vi "WriteEnvironmentInfo.vi"(4 "error in (no error)":errorcluster, 5 "# of Entries (before)":i16, 6 "EnvironmentalInfo":T1, 7 "Pathto FITS Header File":path) -> (0 "error out":errorcluster, 2 "# of Entries (after)":i16, 3 "Path to FITS Header File":path)   [LabVIEW 2015]
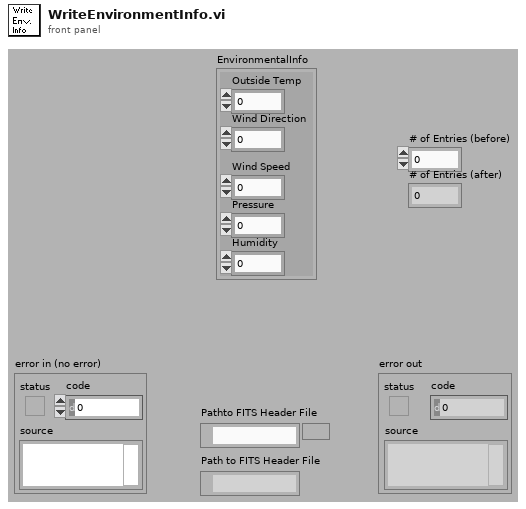
[diagram p1: front panel]
types:
  T1 = cluster{"Outside Temp":dbl, "Wind Direction":dbl, "Wind Speed":dbl, "Pressure":dbl, "Humidity":dbl}
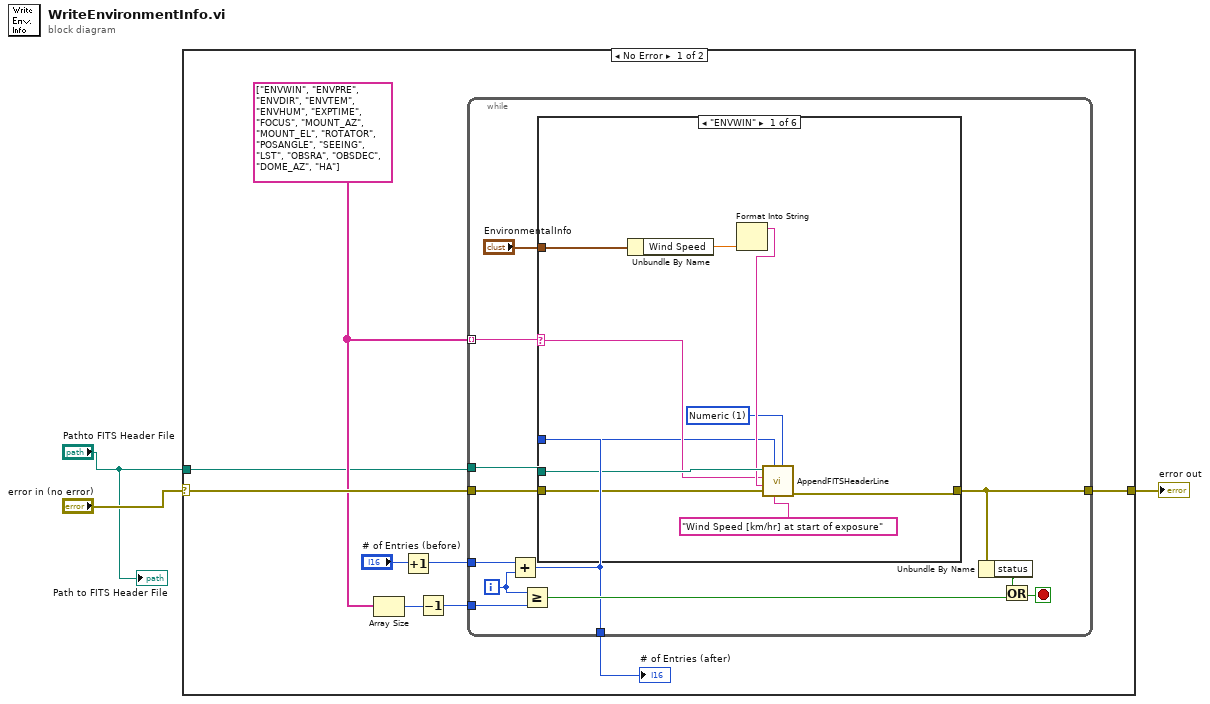
[diagram p0: block diagram]
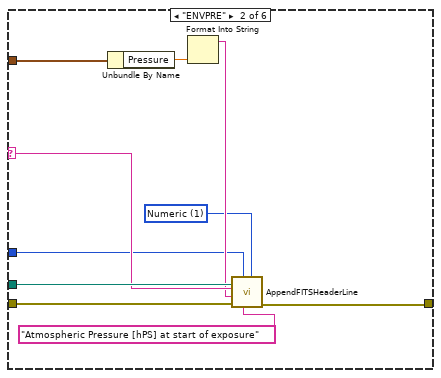
[diagram p2: hidden frame]
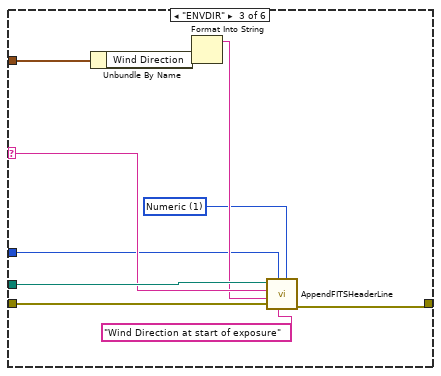
[diagram p3: hidden frame]
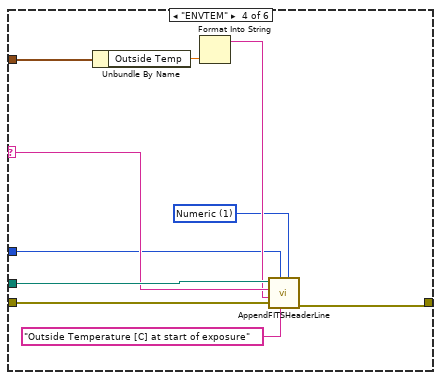
[diagram p4: hidden frame]
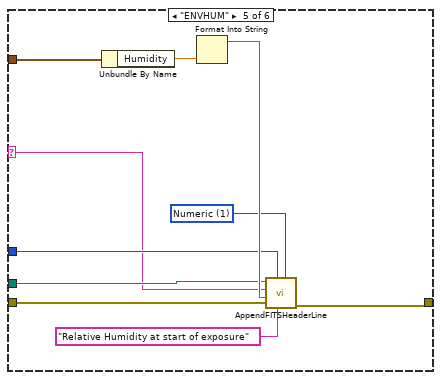
[diagram p5: hidden frame]
diagram:
  n1 = case shown="No Error" "error in (no error)" {
    selector: "error in (no error)" -> [w12 w76]
    tunnel: [w8 w76] -> w2
    tunnel: "Pathto FITS Header File" -> [w7 _]
    frame No Error {
      w11 = string[] ["ENVWIN", "ENVPRE", "ENVDIR", "ENVTEM", "ENVHUM", "EXPTIME", "FOCUS", "MOUNT_AZ", "MOUNT_EL", "ROTATOR", "POSANGLE", "SEEING", "LST", "OBSRA", "OBSDEC", "DOME_AZ", "HA"]
      n2 = Array Size(array=w11) -> (size(s)=w10:i32)
      n3 = Increment(x="# of Entries (before)") -> (x+1=w5:i16)
      n4 = Decrement(x=w10) -> (x-1=w9:i32)
      n5 = while {
        tunnel: w12 -> [w24]
        tunnel: w11 -> [w21] mode=indexing
        tunnel: w9 -> [w20]
        tunnel: [w19] -> w8
        tunnel: w7 -> [w16]
        tunnel: w5 -> [w14]
        tunnel: [w13] -> w4
        i -> [w15]
        stop <- w23 stop-if-true
        n6 = Add(x=w14, y=w15) -> (x+y=w13:i32)
        n7 = Greater Or Equal?(x=w15, y=w20) -> (x >= y?=w18:bool)
        n8 = case shown="\"ENVWIN\"" w21 {
          selector: w21 -> [w28 w40 w49 w59 w66 _]
          tunnel: w24 -> [w32 w43 w52 w62 w69 w75]
          tunnel: [w31 w42 w51 w61 w70 w75] -> w19
          tunnel: "EnvironmentalInfo" -> [w34 w44 w54 w64 w65 _]
          tunnel: w16 -> [w30 w41 w50 w60 w68 _]
          tunnel: w13 -> [w27 w37 w46 w57 w67 _]
          frame "ENVWIN" {
            w26 = u16 1 items=["String", "Numeric", "Boolean"] ("Entry Type")
            n9 = Unbundle By Name(w34) -> ("Wind Speed"=w33:dbl)
            n10 = Format Into String(w33) -> (resulting string=w29:string)  [unwired: 3 in, 1 out]
            n11 = call "AppendFITSHeaderLine.vi"("Entry Type"=w26, "Comment"="Wind Speed [km/hr] at start of exposure", "Entry #"=w27, "error in (no error)"=w32, "Element Value"=w29, "Element Name"=w28, "file path (dialog if empty)"=w30) -> ("error out"=w31:errorcluster)  [unwired: 3 in]
          }
          frame "ENVPRE" {
            w36 = u16 1 items=["String", "Numeric", "Boolean"] ("Entry Type")
            n12 = Unbundle By Name(w44) -> ("Pressure"=w39:dbl)
            n13 = Format Into String(w39) -> (resulting string=w38:string)  [unwired: 3 in, 1 out]
            n14 = call "AppendFITSHeaderLine.vi"("Entry Type"=w36, "Comment"="Atmospheric Pressure [hPS] at start of exposure", "Entry #"=w37, "error in (no error)"=w43, "Element Value"=w38, "Element Name"=w40, "file path (dialog if empty)"=w41) -> ("error out"=w42:errorcluster)  [unwired: 3 in]
          }
          frame "ENVDIR" {
            w47 = u16 1 items=["String", "Numeric", "Boolean"] ("Entry Type")
            n15 = Unbundle By Name(w54) -> ("Wind Direction"=w53:dbl)
            n16 = Format Into String(w53) -> (resulting string=w48:string)  [unwired: 3 in, 1 out]
            n17 = call "AppendFITSHeaderLine.vi"("Entry Type"=w47, "Comment"="Wind Direction at start of exposure", "Entry #"=w46, "error in (no error)"=w52, "Element Value"=w48, "Element Name"=w49, "file path (dialog if empty)"=w50) -> ("error out"=w51:errorcluster)  [unwired: 3 in]
          }
          frame "ENVTEM" {
            w56 = u16 1 items=["String", "Numeric", "Boolean"] ("Entry Type")
            n18 = Unbundle By Name(w64) -> ("Outside Temp"=w63:dbl)
            n19 = Format Into String(w63) -> (resulting string=w58:string)  [unwired: 3 in, 1 out]
            n20 = call "AppendFITSHeaderLine.vi"("Entry Type"=w56, "Comment"="Outside Temperature [C] at start of exposure", "Entry #"=w57, "error in (no error)"=w62, "Element Value"=w58, "Element Name"=w59, "file path (dialog if empty)"=w60) -> ("error out"=w61:errorcluster)  [unwired: 3 in]
          }
          frame "ENVHUM" {
            w72 = u16 1 items=["String", "Numeric", "Boolean"] ("Entry Type")
            n21 = Unbundle By Name(w65) -> ("Humidity"=w74:dbl)
            n22 = Format Into String(w74) -> (resulting string=w73:string)  [unwired: 3 in, 1 out]
            n23 = call "AppendFITSHeaderLine.vi"("Entry Type"=w72, "Comment"="Relative Humidity at start of exposure", "Entry #"=w67, "error in (no error)"=w69, "Element Value"=w73, "Element Name"=w66, "file path (dialog if empty)"=w68) -> ("error out"=w70:errorcluster)  [unwired: 3 in]
          }
          frame "", Default {
          }
        }
        n24 = Unbundle By Name(w19) -> ("status"=w17:bool)
        n25 = Or(x=w17, y=w18) -> (x .or. y?=w23:bool)
      }
      "# of Entries (after)" <- w4
    }
    frame Error {
    }
  }
  "error out" <- w2
  "Path to FITS Header File" <- "Pathto FITS Header File"
